vi "Examen.vi"() -> ()   [LabVIEW 2020]
uses:
  <vilib>/numeric/Random Number (Range) U64.vi
  <vilib>/numeric/sub_Random U32.vi
panel:
  out "Saving Data":bool
  in  "stop":bool
  out "numero de muestras":dbl
  out "tabla":string[][](array[string])
  out "dentro del rango":bool
  in  "Max":dbl
  in  "Min":dbl
  out "Histeresis":bool
  out "Numeros aleatorios sin filtro":u64
  out "Filtro Ema":dbl(graph)
  out "Numeros Aleatorios y filtro EMA":cluster{"number":u64, dbl}[](graph)
  out "Valores aleatorios":u64(graph)
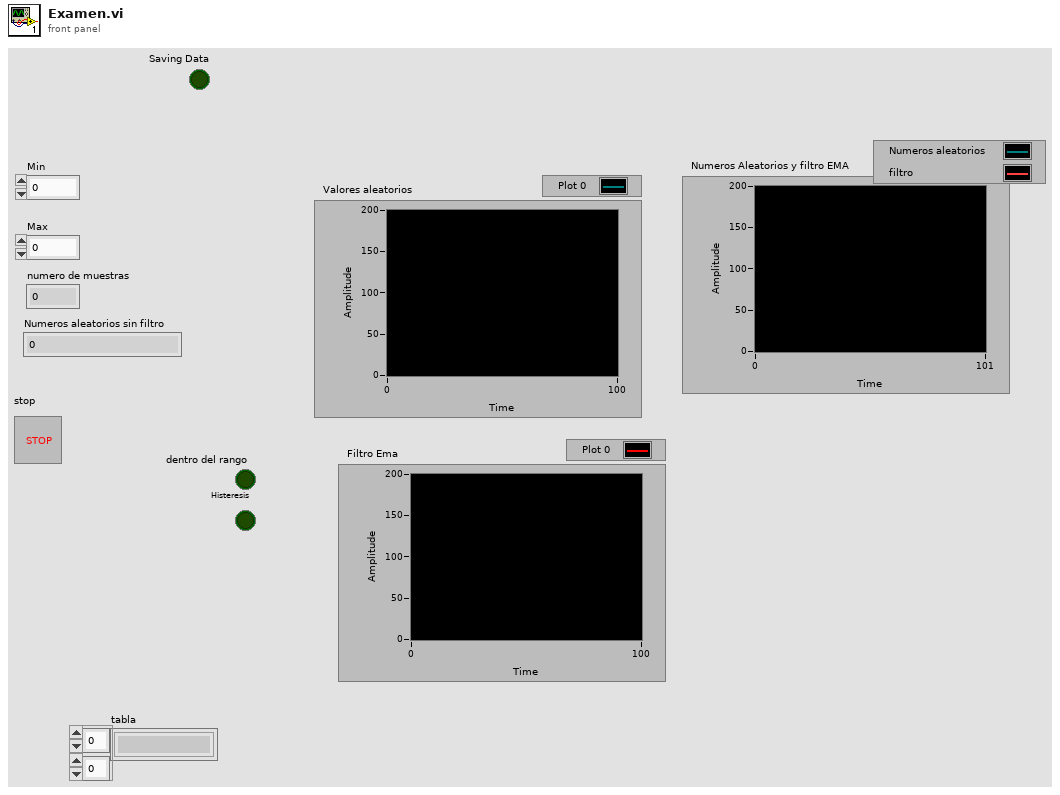
[diagram p1: front panel]
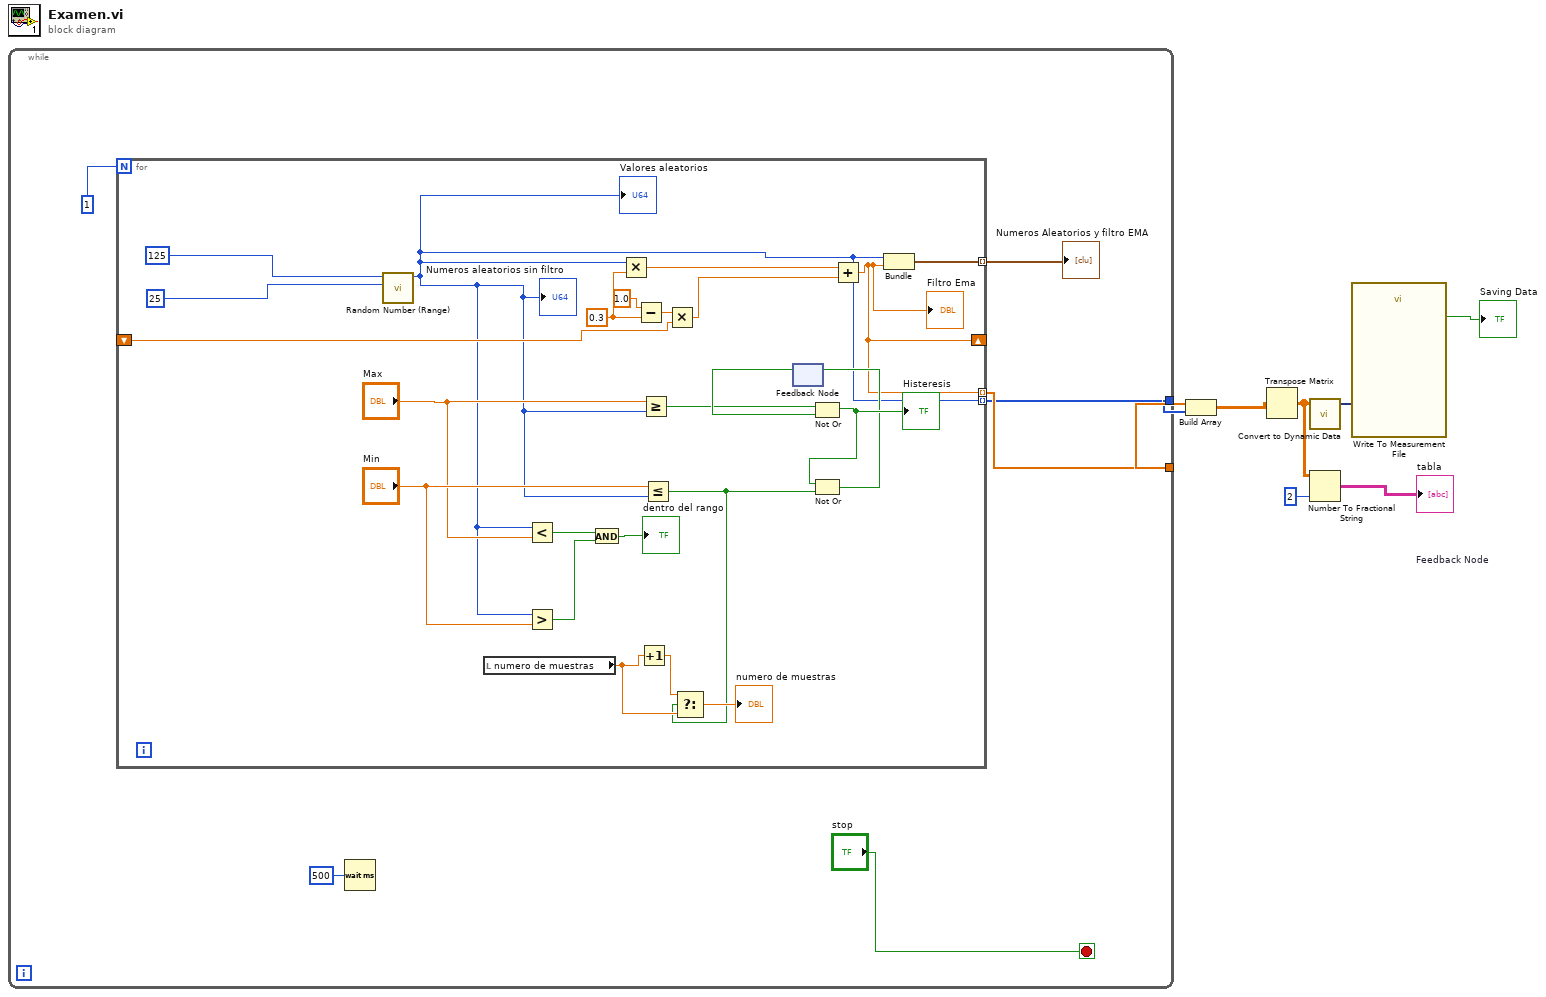
[diagram p0: block diagram]
diagram:
  n1 = while {
    tunnel: [w12] -> w4
    tunnel: [w11] -> w3
    stop <- "stop" stop-if-true
    n2 = for {
      N: 1 -> [_]
      shift-right: [w25] -> _
      shift-left: _ -> [w33]
      tunnel: [w32] -> w13 mode=indexing
      tunnel: [w25] -> w12 mode=indexing
      tunnel: [w18] -> w11 mode=indexing
      w37 = 0.3 ("y")
      n3 = call-poly <vilib>:"Random Number (Range).vi"("lower bound (0)"=u64 25, "upper bound (100)"=u64 125) -> ("number"=w18:u64)  [unwired: 9 in]
      "Numeros aleatorios sin filtro" <- w18
      "Valores aleatorios" <- w18
      n4 = local read "numero de muestras"() -> (w19:dbl)
      n5 = Less?(x=w18, y="Max") -> (x < y?=w17:bool)
      n6 = Greater?(x=w18, y="Min") -> (0:w28:bool)
      n7 = And(x=w17, y=w28) -> (x .and. y?=→"dentro del rango":bool)
      n8 = Multiply(x=w18, y=w37) -> (x*y=w35:dbl)
      n9 = Subtract(x=1.0, y=w37) -> (x-y=w36:dbl)
      n10 = Increment(x=w19) -> (x+1=w20:dbl)
      n11 = Greater Or Equal?(x="Max", y=w18) -> (x >= y?=w16:bool)
      n12 = Less Or Equal?(x="Min", y=w18) -> (x <= y?=w15:bool)
      n13 = Multiply(x=w36, y=w33) -> (x*y=w34:dbl)
      n14 = Select(t=w20, s=w15, f=w19) -> (s? t:f=→"numero de muestras":dbl)
      n15 = feedback #1 "Feedback Node"() -> (w30:bool)  [unwired: 1 in]
      n16 = Not Or(1:w30, 2:w16) -> (0:w31:bool)
      "Histeresis" <- w31
      n17 = Not Or(1:w15, 2:w31) -> (0:w29:bool)
      n18 = feedback-in #1(w29) -> ()
      n19 = Add(x=w35, y=w34) -> (x+y=w25:dbl)
      "Filtro Ema" <- w25
      n20 = Bundle("number"=w18, w25) -> (w32:cluster{"number":u64, dbl})  [unwired: 1 in]
    }
    "Numeros Aleatorios y filtro EMA" <- w13
    n21 = Wait (ms)(milliseconds to wait=u32 500) -> ()  [unwired: 1 out]
  }
  n22 = Build Array(w4, w3) -> (w8:dbl[][])
  n23 = Transpose Matrix(1:w8) -> (0:w5:dbl[][])
  n24 = call "Convert to Dynamic Data"("2D Array"=w5) -> ("Dynamic Data Type"=w6:dynamicdata)  [unwired: 3 in]
  n25 = Number To Fractional String(number=w5, precision (6)=i16 2) -> (F-format string=→"tabla":string[][])  [unwired: 2 in]
  n26 = call "Write To Measurement File"("Signals"=w6) -> ("Saving Data"=→"Saving Data":bool)  [unwired: 16 in, 2 out]
